vi "4461 - Create IO Channels Parallel Uneven.vi"(8 "error in":errorcluster, 11 "Lockin":refnum<class "Instrument.Lockin.lvclass">) -> (0 "error out":errorcluster, 3 "Instrument.Lockin out":refnum<class "Instrument.Lockin.lvclass">)   [LabVIEW 2016, in "Instrument.Lockin.lvclass"]
uses:
  Instrument.Lockin.lvclass
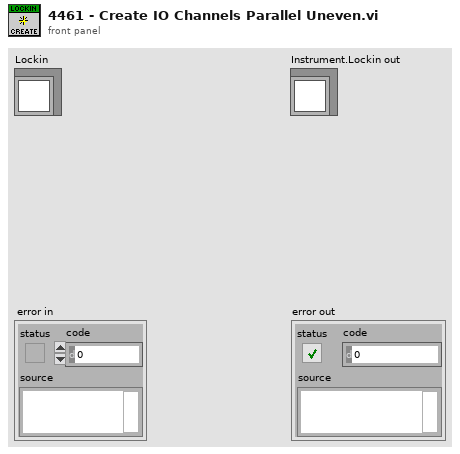
[diagram p1: front panel]
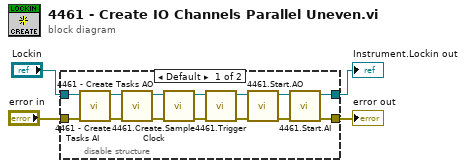
[diagram p0: block diagram]
diagram:
  n1 = disable-structure shown="Default" {
    disable-tunnel: "Lockin" -> [w8 w20]
    disable-tunnel: "error in" -> [w7 w19]
    disable-tunnel: [w6 w20] -> w2
    disable-tunnel: [w5 w19] -> w1
    frame condition #0 (active) {
      n2 = call "4461 - Create Tasks AI.vi"("error in (no error)"=w7, "Instrument.Lockin in"=w8) -> ("error out"=w9:errorcluster, "Instrument.Lockin out"=w10:refnum<class "Instrument.Lockin.lvclass">)  [unwired: 8 in]
      n3 = call "4461 - Create Tasks AO.vi"("error in (no error)"=w9, "Instrument.Lockin in"=w10) -> ("error out"=w11:errorcluster, "Instrument.Lockin out"=w12:refnum<class "Instrument.Lockin.lvclass">)  [unwired: 8 in]
      n4 = call "4461.Create.Sample Clock.vi"("error in (no error)"=w11, "Instrument.Lockin in"=w12) -> ("error out"=w13:errorcluster, "Instrument.Lockin out"=w14:refnum<class "Instrument.Lockin.lvclass">)  [unwired: 8 in]
      n5 = call "4461.Trigger.vi"("error in (no error)"=w13, "Instrument.Lockin in"=w14) -> ("error out"=w18:errorcluster, "Instrument.Lockin out"=w15:refnum<class "Instrument.Lockin.lvclass">)  [unwired: 8 in]
      n6 = call "4461.Start.AO.vi"("error in (no error)"=w18, "Instrument.Lockin in"=w15) -> ("error out"=w17:errorcluster, "Instrument.Lockin out"=w16:refnum<class "Instrument.Lockin.lvclass">)  [unwired: 8 in]
      n7 = call "4461.Start.AI.vi"("error in (no error)"=w17, "Instrument.Lockin in"=w16) -> ("error out"=w5:errorcluster, "Instrument.Lockin out"=w6:refnum<class "Instrument.Lockin.lvclass">)  [unwired: 6 in]
    }
    frame condition #1 {
    }
  }
  "error out" <- w1
  "Instrument.Lockin out" <- w2
